vi "CenterBack.vi"(0 "Our Robot in":T3={"id"=0, "function"=enum."Attacker", "x"=0.0, "y"=0.0, "orientation"=0.0, "v_tangent"=0.0, "v_normal"=0.0, "v_ang"=0.0, "kick_x"=0.0, "kick_z"=0.0, "dribble"=FALSE, "Timestamp"=timestamp(0 s since 1904-01-01), "estimatives"={"est_v_tangent"=0.0, "est_v_normal"=0.0, "est_vx"=0.0, "est_vy"=0.0, "Pos Robot Est"=[]}, "dest_x_kick"=0.0, "dest_y_kick"=0.0, "Gap Coord"=[], "States"=enum."GoToTangent", "Path "=[], "Path  Smooth"=[], "Dest"=[]}, 1 "total":i32, 2 "Id duelist":u32, 3 "Stop?":bool, 4 "AI Parameters":T1={"GotoKick"={"Dist do cone a frente"=150.0, "attacker farback"=1500.0, "Perto"=300.0, "min dist to kick"=150.0, "kick eps"=0.05, "Time to transition"=0.0}, "Attacker"={"CC chute"=0.09, "CC passe"=0.045, "Kick Force"=100.0, "ball-robot Kick"=200.0, "ball-robot Pass"=0.3, "drible\nAttk"=FALSE}, "Defender"={"D max"=1700.0, "Vel p/ robô av"=1000.0, "Kick Force"=100.0, "D atk-def"=0.0, "D farback"=0.0, "drible\ndef"=FALSE, "drible\ngoalie"=FALSE}, "Timeout"={"Field/v in x"=6.0, "Dist Robots"=300, "Dist up in y"=300}, "Pose Striker"={"dist"=200.0, "Numeric"=-4.0, "dist 2"=200.0, "drible\nstriker"=FALSE}, "Dist Stop"=300.0, "D ball out"=200, "D central gap "=150.0, "T pass"=0.0, "Force ++"=0.0, "range kick"=0.0, "Chute alto"=TRUE, "Marcador novo"=TRUE, "drible"=FALSE, "D drible"=300.0, "Versão Striker"=enum."Auto", "Defesa"=enum."ManMark", "Marcador"=enum."Marcar Segundo mais perigoso", "Receptor passe"=enum."Auto", "Área"=enum."Quadrada", "Decisão\nsimples?"=FALSE} {"D drible" format="%#_13g"; "D central gap" format="%#_13g"; "Dist Stop" format="%#_13g"; "Pose Striker"."Numeric" format="%#_13g"; "Defender"."Kick Force" format="%#_13g"; "Defender"."Vel p/ robô av" format="%#_13g"; "Attacker"."ball-robot Kick" format="%#_13g"; "Attacker"."Kick Force" format="%#_13g"; "Attacker"."CC passe" format="%#_13g"; "Attacker"."CC chute" format="%#_13g"; "GotoKick"."kick eps" format="%#_13g"; "GotoKick"."min dist to kick" format="%#_13g"; "GotoKick"."Perto" format="%#_13g"; "GotoKick"."attacker farback" format="%#_13g"; "GotoKick"."Dist do cone a frente" format="%#_13g"}, 5 "balls":T8[](array[typedef]), 7 "Dribble":bool=TRUE, 9 "Field Size in":T9, 10 "Atacando contra?":bool=TRUE, 11 "Field defense":dbl[](array[numeric]), 12 "Defensores":u32[](array[numeric]), 14 "IA State Input 2":T2={"our_robots"=[], "enemy_robots"=[], "balls"=[], "geometry"={"line_width"=0, "field_length"=0, "field_width"=0, "boundary_width"=0, "referee_width"=0, "goal_width"=0, "goal_depth"=0, "goal_wall_width"=0, "center_circle_radius"=0, "defense_radius"=0, "defense_stretch"=0, "free_kick_from_defense_dist"=0, "penalty_spot_from_field_line_dist"=0, "penalty_line_from_spot_dist"=0}, "IA Judge"={"stage"="", "command"="", "our_goalie_id"=0.0, "enemy_goalie_id"=0.0, "command enum"=enum."Halt", "Time"=enum."Azul"}, "Received Timestamp"=timestamp(0 s since 1904-01-01), "Events"={"Touch"=FALSE, "Ball out"=FALSE, "id touch"=0.0, "Ball out of \nVision"=FALSE, "Ball inside \nGoalie area"=FALSE, "Robot not responding"=FALSE, "Robots responding status"=[1.0, 1.0, 1.0, 1.0, 1.0, 1.0], "Enemy Ball \nPossession"=FALSE, "Pass State"=FALSE, "id end of pass"=0.0, "Kick"=FALSE, "Id ini Possession"=0.0, "Ball Possesion"=FALSE, "Id Possesion"=0.0, "Direct Kick"=FALSE, "2nd Strk Ativo"=FALSE}}) -> (6 "Robot out":T3={"id"=0, "function"=enum."Attacker", "x"=0.0, "y"=0.0, "orientation"=0.0, "v_tangent"=0.0, "v_normal"=0.0, "v_ang"=0.0, "kick_x"=0.0, "kick_z"=0.0, "dribble"=FALSE, "Timestamp"=timestamp(0 s since 1904-01-01), "estimatives"={"est_v_tangent"=0.0, "est_v_normal"=0.0, "est_vx"=0.0, "est_vy"=0.0, "Pos Robot Est"=[]}, "dest_x_kick"=0.0, "dest_y_kick"=0.0, "Gap Coord"=[], "States"=enum."GoToTangent", "Path "=[], "Path  Smooth"=[], "Dest"=[]}, 8 "Pos Centers Back":dbl[][](array[numeric]), 13 "Zageuiro duelist?":bool=TRUE)   [LabVIEW 2018]
uses:
  Core/AI Robot.ctl
  Functions Enum.ctl
  AttackerStates.ctl
  Path Planning/RRT/PathDests.ctl
  Path Planning/RRT/PathDest.ctl
  Core/AI Ball.ctl
  Core/Field Size.ctl
  Core/AI Input.ctl
  Core/AI Judge.ctl
  Command Enum.ctl
  Util/Events/Events.ctl
  AI Parameters.ctl
  PersonalityEnum.ctl
  <vilib>/Analysis/_algsub.llb/Real Vector Norm.vi
  <vilib>/Analysis/NI_AALPro.lvlib
panel:
  in  "element":dbl=-2000.0 format="%#_13g"
  in  "dist to defender\nattacker evasion":dbl=200.0
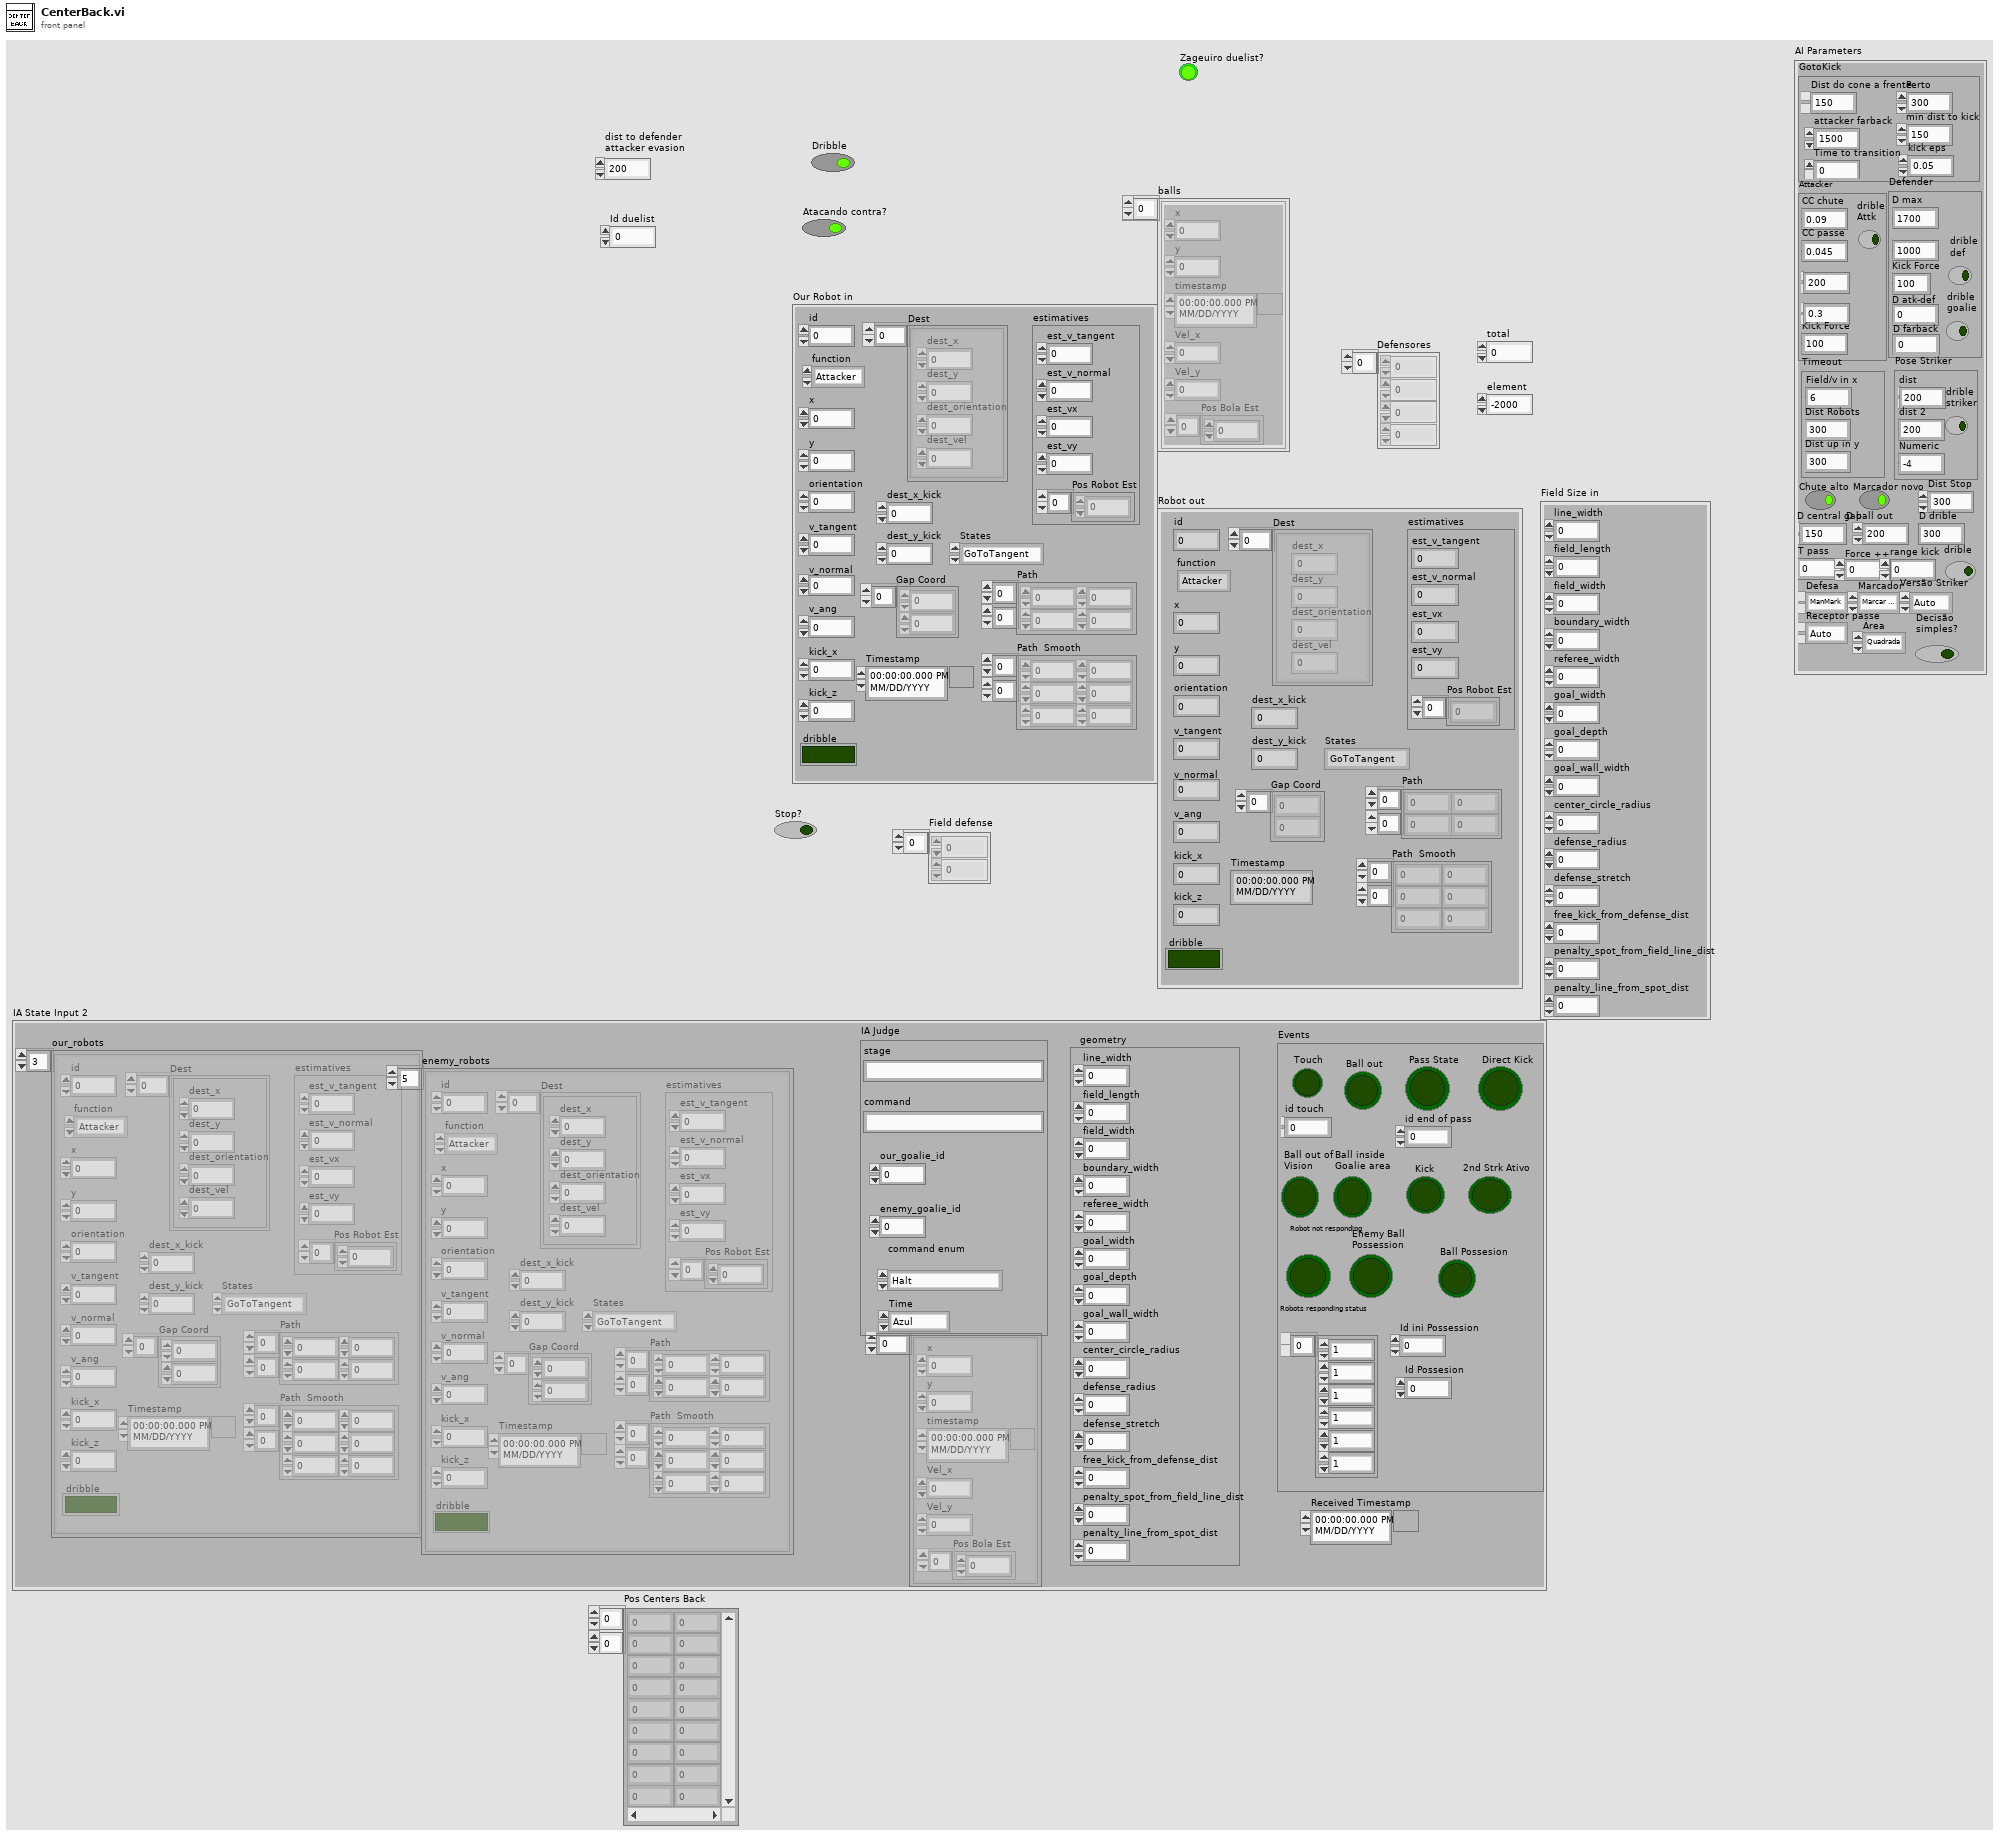
[diagram p1: front panel]
types:
  T1 = typedef "AI Parameters.ctl" = cluster{"GotoKick":cluster{"Dist do cone a frente":dbl, "attacker farback":dbl, "Perto":dbl, "min dist to kick":dbl, "kick eps":dbl, "Time to transition":dbl}, "Attacker":cluster{"CC chute":dbl, "CC passe":dbl, "Kick Force":dbl, "ball-robot Kick":dbl, "ball-robot Pass":dbl, "drible\nAttk":bool}, "Defender":cluster{"D max":dbl, "Vel p/ robô av":dbl, "Kick Force":dbl, "D atk-def":dbl, "D farback":dbl, "drible\ndef":bool, "drible\ngoalie":bool}, "Timeout":cluster{"Field/v in x":dbl, "Dist Robots":u32, "Dist up in y":u32}, "Pose Striker":cluster{"dist":dbl, "Numeric":dbl, "dist 2":dbl, "drible\nstriker":bool}, "Dist Stop":dbl, "D ball out":i32, "D central gap ":dbl, "T pass":dbl, "Force ++":dbl, "range kick":dbl, "Chute alto":bool, "Marcador novo":bool, "drible":bool, "D drible":dbl, "Versão Striker":enum16{"Auto", "3", "2", "1"}, "Defesa":enum16{"ManMark", "Barreira"}, "Marcador":enum16{"Marcar Segundo mais perigoso", "Marcar o mais perigoso"}, "Receptor passe":enum16{"Auto", "2nd Striker", "Striker"}, "Área":enum16{"Quadrada", "Circular"}, "Decisão\nsimples?":bool}
  T2 = typedef "AI Input.ctl" = cluster{"our_robots":T3[], "enemy_robots":T3[], "balls":T8[], "geometry":T9, "IA Judge":T10, "Received Timestamp":timestamp, "Events":T12}
  T3 = typedef "AI Robot.ctl" = cluster{"id":u32, "function":T4, "x":dbl, "y":dbl, "orientation":dbl, "v_tangent":dbl, "v_normal":dbl, "v_ang":dbl, "kick_x":dbl, "kick_z":dbl, "dribble":bool, "Timestamp":timestamp, "estimatives":cluster{"est_v_tangent":dbl, "est_v_normal":dbl, "est_vx":dbl, "est_vy":dbl, "Pos Robot Est":dbl[]}, "dest_x_kick":dbl, "dest_y_kick":dbl, "Gap Coord":dbl[], "States":T5, "Path ":dbl[][], "Path  Smooth":dbl[][], "Dest":T6}
  T4 = typedef "Functions Enum.ctl" = enum16{"2nd Striker", "Attacker", "Goalie", "Defender", "Striker", "Goto 0", "Dummy", "Kicker", "ZigZag 0", "ZigZag 1", "ZigZag 2", "ZigZag 3", "ZigZag 4", "ZigZag 5", "ZigZag 6", "ZigZag 7", "ZigZag 8", ""}
  T5 = typedef "AttackerStates.ctl" = enum16{"Pass", "GoToTangent", "BallGetting", "GoToKick", ""}
  T6 = typedef "PathDests.ctl" = T7[]
  T7 = typedef "PathDest.ctl" = cluster{"dest_x":dbl, "dest_y":dbl, "dest_orientation":dbl, "dest_vel":dbl}
  T8 = typedef "AI Ball.ctl" = cluster{"x":dbl, "y":dbl, "timestamp":timestamp, "Vel_x":dbl, "Vel_y":dbl, "Pos Bola Est":dbl[]}
  T9 = typedef "Field Size.ctl" = cluster{"line_width":u32, "field_length":u32, "field_width":u32, "boundary_width":u32, "referee_width":u32, "goal_width":u32, "goal_depth":u32, "goal_wall_width":u32, "center_circle_radius":u32, "defense_radius":u32, "defense_stretch":u32, "free_kick_from_defense_dist":u32, "penalty_spot_from_field_line_dist":u32, "penalty_line_from_spot_dist":u32}
  T10 = typedef "AI Judge.ctl" = cluster{"stage":string, "command":string, "our_goalie_id":dbl, "enemy_goalie_id":dbl, "command enum":T11, "Time":enum16{"Azul", "Amarelo"}}
  T11 = typedef "Command Enum.ctl" = enum16{"Halt", "Stop", "Force Start", "PKA Normal Start", "Prepare Kickoff Ally", "PKE Normal Start", "Prepare Kickoff Enemy", "Prepare Penalty Ally", "PPA Normal Start", "Prepare Penalty Enemy", "PPE Normal Start", "Direct Free Enemy", "Direct Free Ally", "Indirect Free Enemy", "Indirect Free Ally", "Timeout Enemy", "Timeout Ally", "Goal Enemy", "Goal Ally", "Ball Placement Enemy", "Ball Placement Ally", "Normal Half Time", "Extra Time Break", "Extra Half Time", "None", "Post Game"}
  T12 = typedef "Events.ctl" = cluster{"Touch":bool, "Ball out":bool, "id touch":dbl, "Ball out of \nVision":bool, "Ball inside \nGoalie area":bool, "Robot not responding":bool, "Robots responding status":dbl[], "Enemy Ball \nPossession":bool, "Pass State":bool, "id end of pass":dbl, "Kick":bool, "Id ini Possession":dbl, "Ball Possesion":bool, "Id Possesion":dbl, "Direct Kick":bool, "2nd Strk Ativo":bool}
  T13 = cluster{"D max":dbl, "Vel p/ robô av":dbl, "Kick Force":dbl, "D atk-def":dbl, "D farback":dbl, "drible\ndef":bool, "drible\ngoalie":bool}
  T14 = typedef "PersonalityEnum.ctl" = enum16{"Attacker", "Striker", "Defender", "Goalie"}
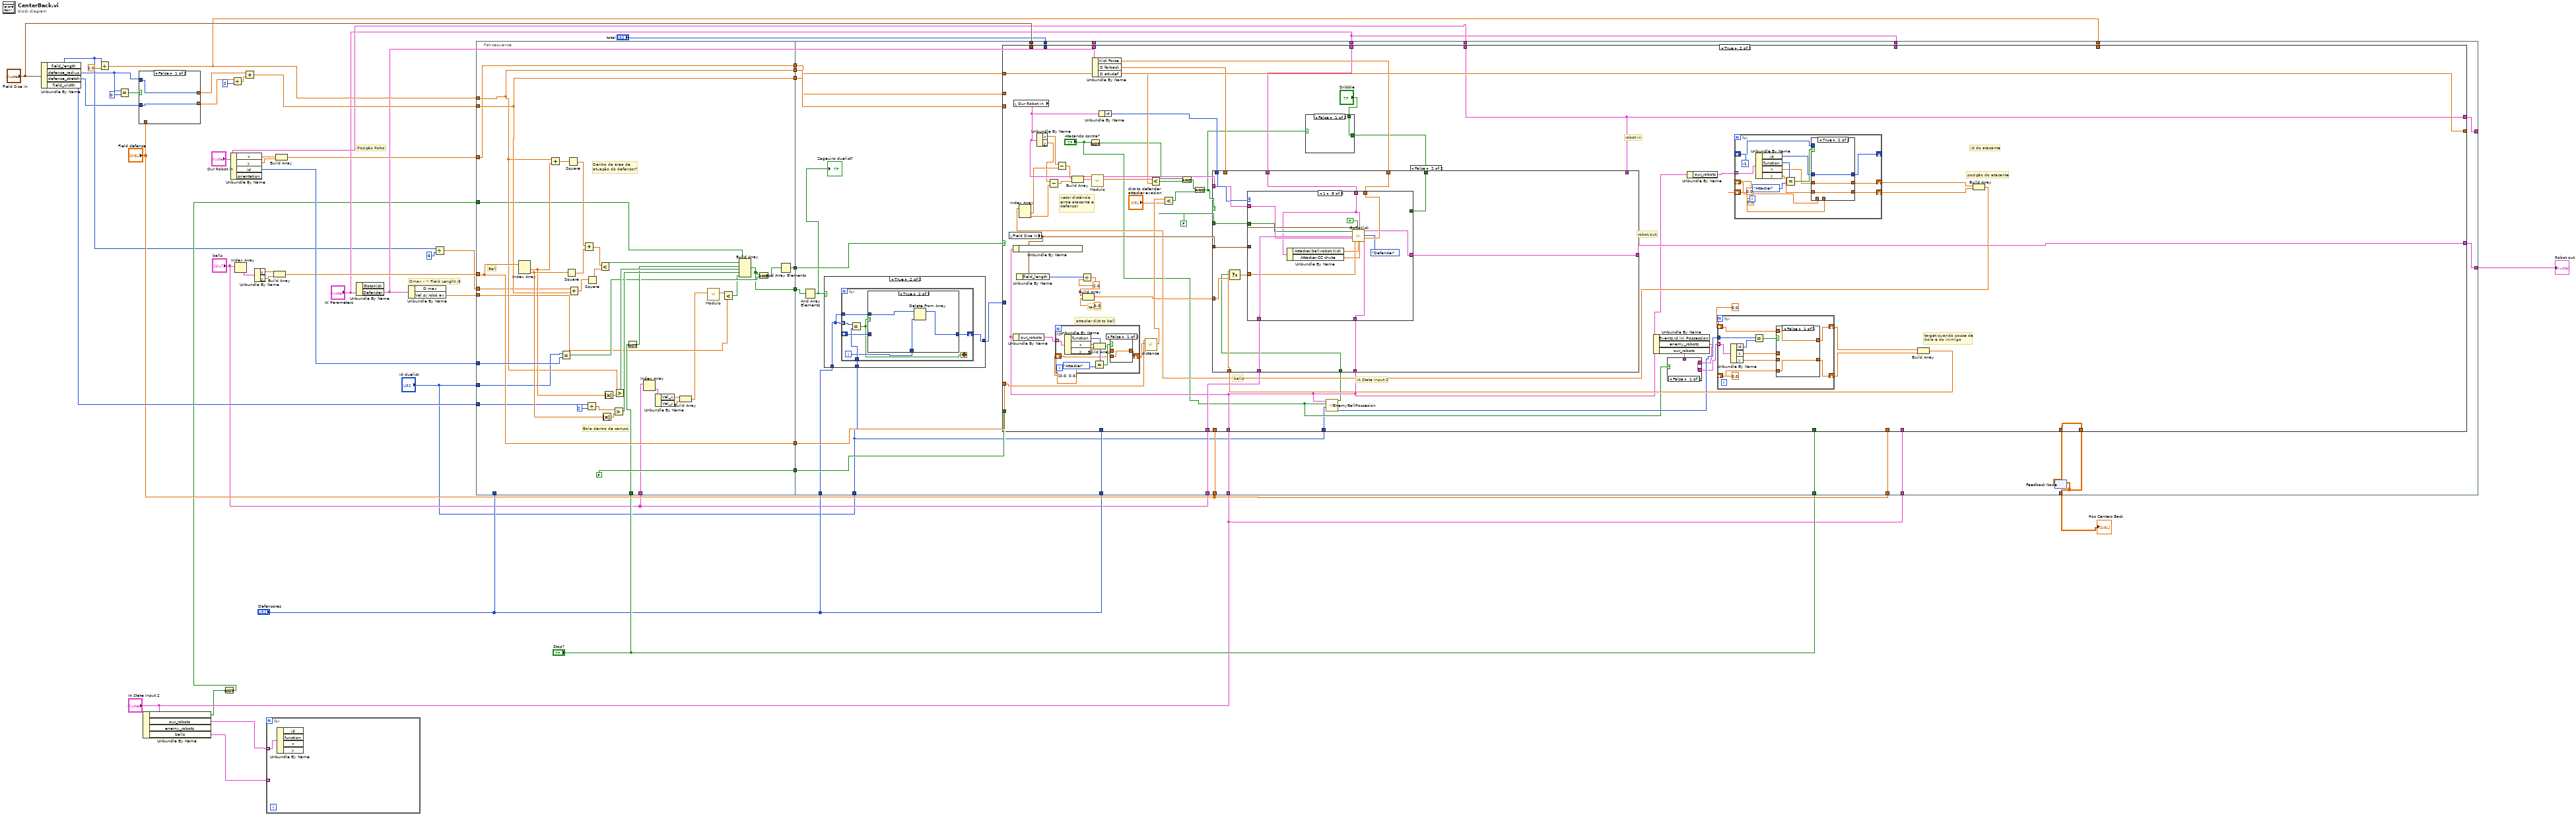
[diagram p0: block diagram]
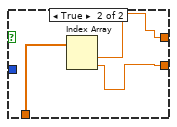
[diagram p2: hidden frame]
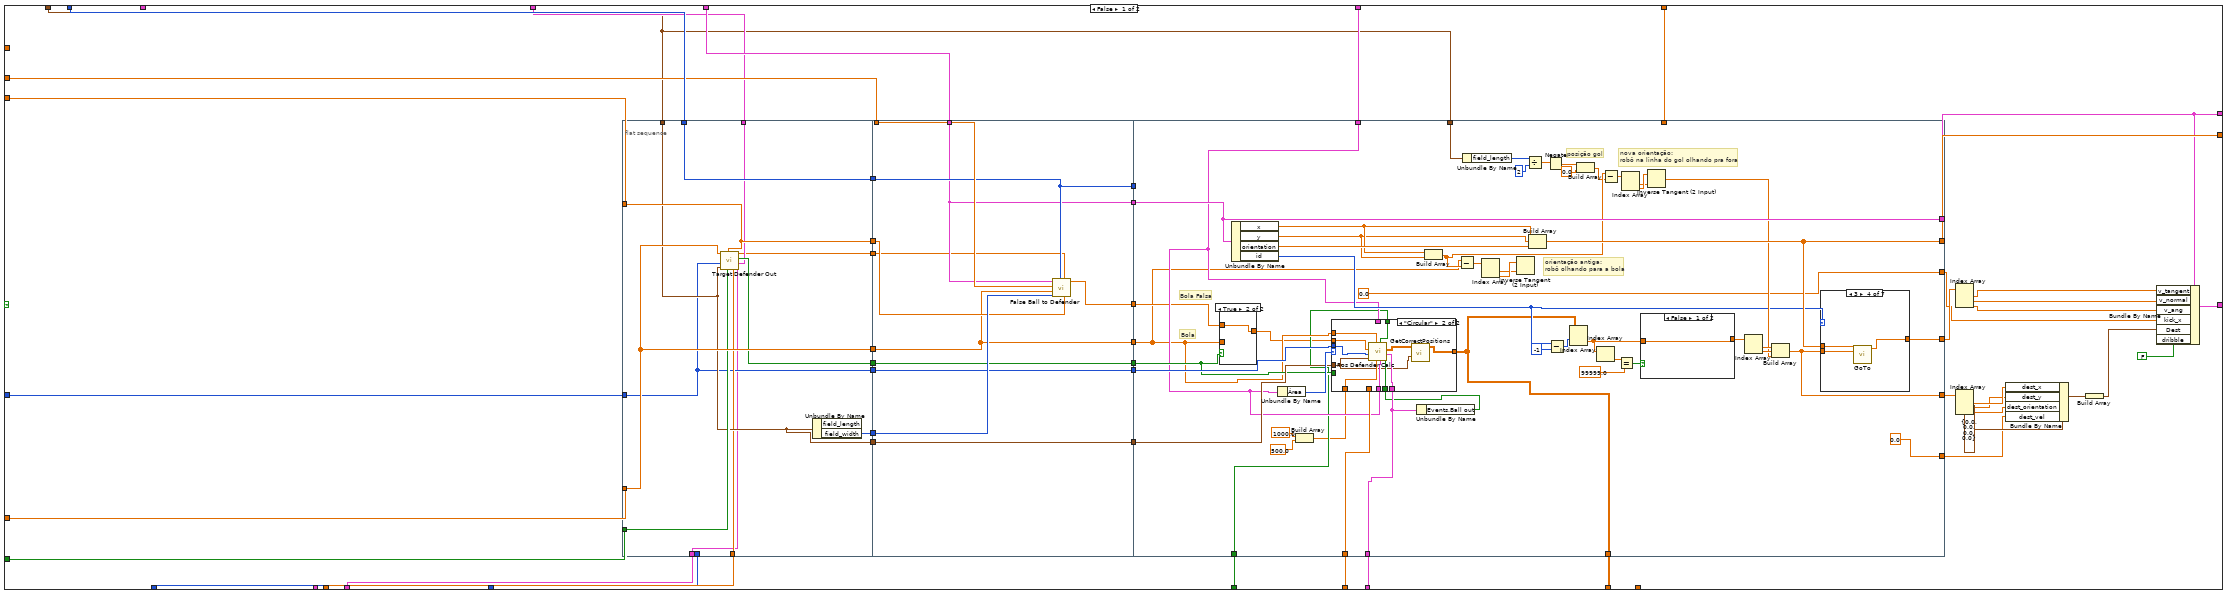
[diagram p5: hidden frame]
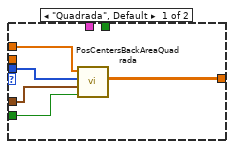
[diagram p6: hidden frame]
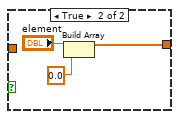
[diagram p7: hidden frame]
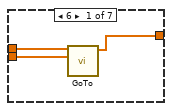
[diagram p8: hidden frame]
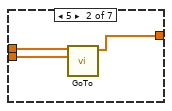
[diagram p9: hidden frame]
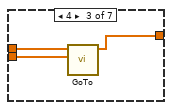
[diagram p10: hidden frame]
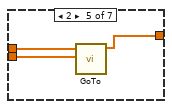
[diagram p11: hidden frame]
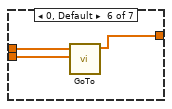
[diagram p12: hidden frame]
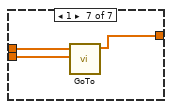
[diagram p13: hidden frame]
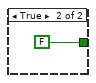
[diagram p15: hidden frame]
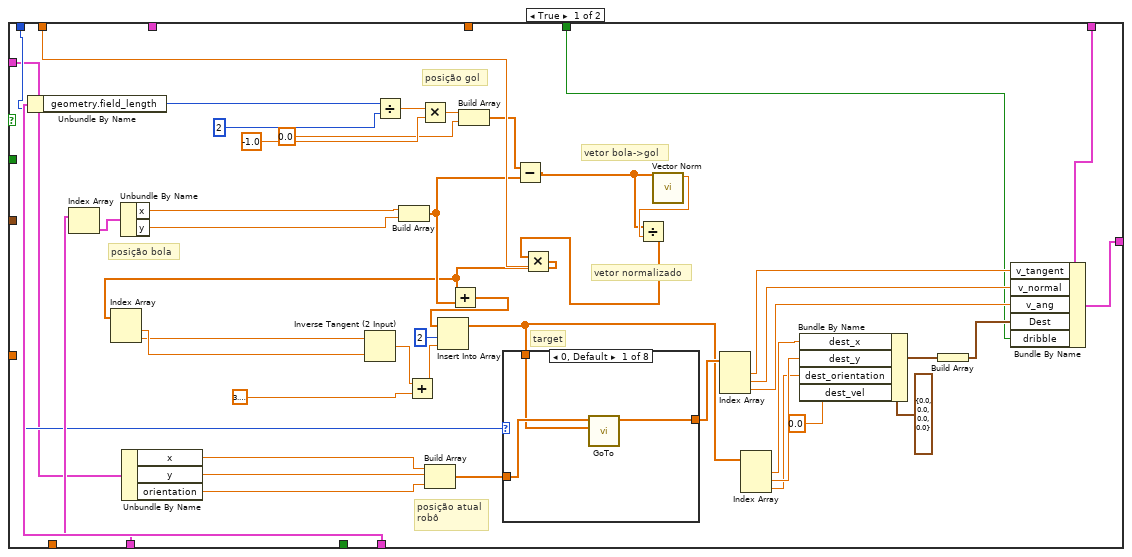
[diagram p18: hidden frame]
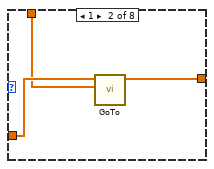
[diagram p19: hidden frame]
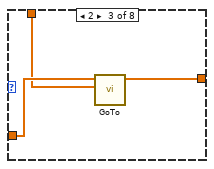
[diagram p20: hidden frame]
diagram:
  # "Dmax - > Field Lenght /6"
  # "Posição Robo"
  n1 = Unbundle By Name("Field Size in") -> ("field_length"=w3:u32, "defense_radius"=w28:u32, "defense_stretch"=w27:u32, "field_width"=w41:u32)
  n2 = Divide(x=w3, y=2.0) -> (x/y=w19:dbl)
  n3 = Equal?(x=w28, y=u32 0) -> (x = y?=w26:bool)
  n4 = case shown="False" w26 {
    tunnel: [w50 w52] -> w25
    tunnel: w28 -> [w50 _]
    tunnel: w27 -> [w49 _]
    tunnel: [w49 w51] -> w24
    tunnel: "Field defense" -> [_ w53]
    frame False {
    }
    frame True {
      n5 = Index Array(array=w53) -> (element #1=w52:dbl, element #2=w51:dbl)  [unwired: 2 in]
    }
  }
  n6 = Unbundle By Name("IA State Input 2") -> ("Events.Ball inside \nGoalie area"=w5:bool, "our_robots"=w10:T3[], "balls"=w9:T8[])  [unwired: 1 out]
  n7 = Not(x=w5) -> (.not. x?=w4:bool)
  n8 = Unbundle By Name("Our Robot in") -> ("x"=w38:dbl, "y"=w37:dbl, "id"=w42:u32)  [unwired: 1 out]
  n9 = Divide(x=w24, y=u32 2) -> (x/y=w47:dbl)
  n10 = Index Array(array="balls") -> (element=w48:T8)  [unwired: 1 in]
  n11 = Add(x=w25, y=w47) -> (x+y=w43:dbl)
  n12 = Unbundle By Name(w48) -> ("x"=w45:dbl, "y"=w12:dbl)
  n13 = for {
    tunnel: w10 -> [w54] mode=indexing
    tunnel: w9 -> [_] mode=indexing
    n14 = Unbundle By Name(w54) -> ()  [unwired: 4 out]
  }
  n15 = Build Array(w45, w12) -> (w20:dbl[])
  n16 = Build Array(w38, w37) -> (w21:dbl[])
  n17 = Unbundle By Name("AI Parameters") -> ("Defender"=w14:T13)  [unwired: 1 out]
  n18 = Unbundle By Name(w14) -> ("Vel p/ robô av"=w15:dbl)  [unwired: 1 out]
  n19 = Divide(x=w3, y=u32 6) -> (x/y=w1:dbl)
  n20 = flat-sequence {
    tunnel: w43 -> [w73]
    tunnel: w19 -> [w72]
    tunnel: w20 -> [w88]
    tunnel: w21 -> [w71]
    tunnel: [w88] -> w36
    tunnel: [w93] -> w35
    tunnel: w42 -> [w92]
    tunnel: w41 -> [w79]
    tunnel: [FALSE ("Target Fora")] -> w34
    tunnel: [w72] -> w33
    tunnel: [w73] -> w32
    tunnel: [w71] -> w31
    tunnel: "Defensores" -> [_]
    tunnel: "Stop?" -> [w70]
    tunnel: [w66] -> w17
    tunnel: "balls" -> [w65]
    tunnel: w1 -> [w62]
    tunnel: w15 -> [w61]
    tunnel: "Id duelist" -> [w56]
    tunnel: w4 -> [w55]
    tunnel: "total" -> [w122]
    tunnel: [w121] -> w8
    tunnel: w36 -> [w120]
    tunnel: w35 -> [w119]
    tunnel: w34 -> [w118]
    tunnel: w33 -> [w116]
    tunnel: "Field Size in" -> [w117]
    tunnel: "Our Robot in" -> [w115]
    tunnel: w32 -> [w114]
    tunnel: [w113] -> _
    tunnel: w31 -> [w112]
    tunnel: "Field defense" -> [w111]
    tunnel: "Field defense" -> [w110]
    tunnel: "Defensores" -> [w109]
    tunnel: "IA State Input 2" -> [w108]
    tunnel: "balls" -> [w107]
    tunnel: "Stop?" -> [w106]
    tunnel: w19 -> [w105]
    tunnel: "Defensores" -> [w104]
    tunnel: w17 -> [w103]
    tunnel: w14 -> [w101]
    tunnel: "AI Parameters" -> [w100]
    tunnel: "AI Parameters" -> [w99]
    tunnel: "IA State Input 2" -> [w98]
    tunnel: [w95] -> w7
    tunnel: "Id duelist" -> [w94]
    frame #0 {
      # "Bola dentro de campo"
      # "Dentro da área de \natuação do defensor?"
      # "Ball"
      n21 = Index Array(array=w88) -> (element #1=w76:dbl, element #2=w80:dbl)  [unwired: 2 in]
      n22 = Add(x=w72, y=w76) -> (x+y=w89:dbl)
      n23 = Equal?(x=w56, y=w92) -> (x = y?=w68:bool)
      n24 = Square(x=w80) -> (x^2=w91:dbl)
      n25 = Square(x=w89) -> (x^2=w90:dbl)
      n26 = Add(x=w62, y=w73) -> (x+y=w75:dbl)
      n27 = Add(x=w90, y=w91) -> (x+y=w85:dbl)
      n28 = Divide(x=w79, y=u32 2) -> (x/y=w82:dbl)
      n29 = Square(x=w75) -> (x^2=w87:dbl)
      n30 = Less?(x=w85, y=w87) -> (x < y?=w86:bool)
      n31 = Absolute Value(x=w80) -> (abs(x)=w81:dbl)
      n32 = Absolute Value(x=w76) -> (abs(x)=w84:dbl)
      n33 = Greater?(x=w82, y=w81) -> (0:w77:bool)
      n34 = Greater?(x=w72, y=w84) -> (0:w83:bool)
      n35 = Not(x=w70) -> (.not. x?=w69:bool)
      n36 = Index Array(array=w65) -> (element=w60:T8)  [unwired: 1 in]
      n37 = Unbundle By Name(w60) -> ("Vel_x"=w59:dbl, "Vel_y"=w58:dbl)
      n38 = Build Array(w59, w58) -> (w57:dbl[])
      n39 = call "Modulo.vi"("2D vector"=w57) -> ("Modulo"=w63:dbl)  [unwired: 10 in]
      n40 = Less?(x=w63, y=w61) -> (x < y?=w64:bool)
      n41 = Build Array(w55, w86, w69, w83, w77, w64) -> (w66:bool[])
      n42 = And(x=w66, y=w68) -> (x .and. y?=w67:bool[])
      n43 = And Array Elements(Boolean array=w67) -> (logical AND=w93:bool)
    }
    frame #1 {
      n44 = And Array Elements(Boolean array=w103) -> (logical AND=w97:bool)
      "Zageuiro duelist?" <- w97
      n45 = case shown="True" w97 {
        tunnel: w104 -> [w123 w125]
        tunnel: [w123 w124] -> w102
        tunnel: w94 -> [_ w126]
        frame False {
        }
        frame True {
          n46 = for {
            tunnel: w125 -> [w133] mode=indexing
            tunnel: w126 -> [w132]
            tunnel: w125 -> [w131]
            shift-right: [w129] -> w124
            shift-left: _ -> [w128]
            i -> [w130]
            stop <- w127 stop-if-true
            n47 = Equal?(x=w133, y=w132) -> (x = y?=w127:bool)
            n48 = case shown="True" w127 {
              tunnel: w131 -> [_ w137]
              tunnel: w130 -> [_ w136]
              tunnel: [w134 w135] -> w129
              tunnel: w128 -> [w134 _]
              frame False {
              }
              frame True {
                n49 = Delete From Array(array=w137, index=w136) -> (array with subset deleted=w135:u32[])  [unwired: 1 in, 1 out]
              }
            }
          }
        }
      }
      n50 = feedback #1() -> (w95:dbl[][])  [unwired: 1 in]
      n51 = case shown="True" w119 {
        tunnel: w122 -> [w186 _]
        tunnel: [w182 w328] -> w121
        tunnel: w120 -> [w181 w321]
        tunnel: w118 -> [w179 _]
        tunnel: w116 -> [w178 _]
        tunnel: w117 -> [w148 _]
        tunnel: w115 -> [w177 w329]
        tunnel: w114 -> [w176 _]
        tunnel: [w162 w363] -> _
        tunnel: [w161 w329] -> w113
        tunnel: w112 -> [_ w363]
        tunnel: w111 -> [w160 _]
        tunnel: w110 -> [w159 _]
        tunnel: w109 -> [w158 _]
        tunnel: w108 -> [w151 w315]
        tunnel: w107 -> [_ w362]
        tunnel: w106 -> [w157 _]
        tunnel: w105 -> [w156 _]
        tunnel: w102 -> [w154 _]
        tunnel: w101 -> [_ w348]
        tunnel: w100 -> [w150 w346]
        tunnel: w99 -> [w153 _]
        tunnel: w98 -> [w152 _]
        tunnel: [w141 w316] -> w96
        tunnel: w95 -> [_ w316]
        tunnel: w94 -> [_ w307]
        frame False {
          n52 = flat-sequence {
            tunnel: w186 -> [w198]
            tunnel: [w199] -> w187
            tunnel: w181 -> [w197]
            tunnel: [w198] -> w180
            tunnel: w179 -> [w195]
            tunnel: w178 -> [w196]
            tunnel: w148 -> [w193]
            tunnel: [w197] -> w175
            tunnel: [w196] -> w174
            tunnel: [w194] -> w170
            tunnel: [w191] -> w167
            tunnel: [w193] -> w165
            tunnel: w159 -> [w192]
            tunnel: w158 -> [_]
            tunnel: w154 -> [w191]
            tunnel: w151 -> [w190]
            tunnel: w150 -> [w189]
            tunnel: [w188] -> w149
            tunnel: w187 -> [w210]
            tunnel: w180 -> [w205]
            tunnel: w177 -> [w202]
            tunnel: w176 -> [w209]
            tunnel: w175 -> [w207]
            tunnel: w174 -> [w208]
            tunnel: [w200] -> w173
            tunnel: [w207] -> w172
            tunnel: [w206] -> w171
            tunnel: w170 -> [w206]
            tunnel: [w205] -> w169
            tunnel: [w204] -> w168
            tunnel: w167 -> [w204]
            tunnel: [w203] -> w166
            tunnel: w165 -> [w203]
            tunnel: [w202] -> w164
            tunnel: w149 -> [w201]
            tunnel: [w254] -> w163
            tunnel: [w253] -> w161
            tunnel: w173 -> [w219]
            tunnel: w172 -> [w218]
            tunnel: w171 -> [w221]
            tunnel: w169 -> [_]
            tunnel: w168 -> [w222]
            tunnel: w166 -> [w223]
            tunnel: w164 -> [w253]
            tunnel: [w250] -> w162
            tunnel: w160 -> [w224]
            tunnel: w157 -> [w215]
            tunnel: w156 -> [_]
            tunnel: [w244] -> w155
            tunnel: w153 -> [w220]
            tunnel: w152 -> [w217]
            tunnel: w148 -> [w243]
            tunnel: [w225] -> w141
            tunnel: [0.0 ("dest_vel")] -> w140
            tunnel: [0.0 ("kick_x")] -> w139
            frame #0 {
              n53 = call "Target Defender Out.vi"("IA State Input"=w190, "AI Parameters"=w189, "Field defense"=w192, "Target Fora in"=w195, "Campo/2"=w196, "Field Size in"=w193, "Defensores"=w191, "Ball"=w197) -> ("Target Fora out"=w194:bool, "Central Position"=w188:dbl[])  [unwired: 2 in]
              n54 = Unbundle By Name(w193) -> ("field_width"=w199:u32)  [unwired: 1 out]
            }
            frame #1 {
              n55 = call "False Ball to Defender.vi"("Campo/2"=w208, "Central Position"=w201, "field_width"=w210, "total"=w205, "Bola"=w207, "raio da área \ndo goleiro"=w209, "Our Robot in"=w202) -> ("Bola Falsa"=w200:dbl[])  [unwired: 4 in]
            }
            frame #2 {
              # "nova orientação:\nrobô na linha do gol olhando pra fora"
              # "orientação antiga:\nrobô olhando para a bola"
              # "posição gol"
              # "Bola"
              # "Bola Falsa"
              n56 = case shown="True" w221 {
                tunnel: [w302 w303] -> w211
                tunnel: w218 -> [w302 _]
                tunnel: w219 -> [_ w303]
                frame False {
                }
                frame True {
                }
              }
              n57 = Unbundle By Name(w253) -> ("x"=w259:dbl, "y"=w258:dbl, "orientation"=w260:dbl, "id"=w229:u32)
              n58 = Unbundle By Name(w220) -> ("Área"=w226:enum16{"Quadrada", "Circular"})
              n59 = Build Array(1000.0, 500.0) -> (w212:dbl[])
              n60 = Unbundle By Name(w217) -> ("Events.Ball out"=w216:bool)
              n61 = case shown="\"Circular\"" w226 {
                tunnel: [w265 w269] -> w225
                tunnel: w224 -> [_ _]
                tunnel: w217 -> [_ w276]
                tunnel: w223 -> [w264 w266]
                tunnel: w222 -> [w263 w273]
                tunnel: w218 -> [w262 w274]
                tunnel: w221 -> [w261 _]
                tunnel: w220 -> [_ _]
                tunnel: w220 -> [_ w275]
                tunnel: w216 -> [_ w272]
                tunnel: w215 -> [_ w271]
                tunnel: w212 -> [_ w268]
                tunnel: w211 -> [_ w267]
                frame "Quadrada", Default {
                  n62 = call "PosCentersBackAreaQuadrada.vi"("Robô fora?"=w261, "geometry"=w264, "Defensores"=w263, "Pos Bola"=w262) -> ("Pos Centers Back"=w265:dbl[][])  [unwired: 6 in, 1 out]
                }
                frame "Circular" {
                  n63 = call "Pos Defender Calc.vi"("Events.Ball out"=w272, "IA State Input"=w276, "AI Parameters"=w275, "Stop?"=w271, "Field defense"=w268, "Real Ball"=w274, "Field Size in"=w266, "Defensores"=w273, "Ball"=w267) -> ("Posição dos Defensores"=w270:dbl[][])  [unwired: 1 in, 1 out]
                  n64 = call "GetCorrectPositions.vi"("Field Size in"=w266, "Posição dos defensores"=w270) -> ("Posição dos defensores correta"=w269:dbl[][])  [unwired: 9 in]
                }
              }
              n65 = Build Array(w259, w258) -> (w237:dbl[])
              n66 = Subtract(x=w218, y=w237) -> (x-y=w257:dbl[])
              n67 = Unbundle By Name(w243) -> ("field_length"=w242:u32)
              n68 = Index Array(array=w257) -> (element #1=w255:dbl, element #2=w256:dbl)  [unwired: 2 in]
              n69 = Inverse Tangent (2 Input)(1:w255, 2:w256) -> ()  [unwired: 1 out]
              n70 = Divide(x=w242, y=u32 2) -> (x/y=w240:dbl)
              n71 = Build Array(w259, w258, w260) -> (w250:dbl[])
              n72 = Negate(x=w240) -> (-x=w239:dbl)
              n73 = Subtract(x=w229, y=-1) -> (x-y=w227:u32)
              n74 = Index Array(array=w225, index (row)=w227) -> (element=w248:dbl[])  [unwired: 1 in]
              n75 = Build Array(w239, 0.0 ("element")) -> (w236:dbl[])
              n76 = Index Array(array=w248) -> (element=w247:dbl)  [unwired: 1 in]
              n77 = Subtract(x=w237, y=w236) -> (x-y=w235:dbl[])
              n78 = Equal?(x=w247, y=99999.0) -> (x = y?=w246:bool)
              n79 = Index Array(array=w235) -> (element #1=w233:dbl, element #2=w234:dbl)  [unwired: 2 in]
              n80 = case shown="False" w246 {
                tunnel: [w277 w279] -> w249
                tunnel: w248 -> [w277 _]
                frame False {
                }
                frame True {
                  n81 = Build Array("element", 0.0 ("element")) -> (w279:dbl[])
                }
              }
              n82 = Inverse Tangent (2 Input)(1:w233, 2:w234) -> (0:w232:dbl)
              n83 = Index Array(array=w249) -> (element #1=w252:dbl, element #2=w251:dbl)  [unwired: 2 in]
              n84 = Build Array(w252, w251, w232) -> (w244:dbl[])
              n85 = case shown="3" w229 {
                tunnel: [w281 w284 w287 w290 w293 w296 w299] -> w254
                tunnel: w244 -> [w282 w286 w288 w291 w294 w297 w300]
                tunnel: w250 -> [w283 w285 w289 w292 w295 w298 w301]
                frame 6 {
                  n86 = call "GoTo.vi"("Target"=w282, "Position"=w283) -> ("Output\nVelocity"=w281:dbl[])  [unwired: 8 in, 1 out]
                }
                frame 5 {
                  n87 = call "GoTo.vi"("Target"=w286, "Position"=w285) -> ("Output\nVelocity"=w284:dbl[])  [unwired: 8 in, 1 out]
                }
                frame 4 {
                  n88 = call "GoTo.vi"("Target"=w288, "Position"=w289) -> ("Output\nVelocity"=w287:dbl[])  [unwired: 8 in, 1 out]
                }
                frame 3 {
                  n89 = call "GoTo.vi"("Target"=w291, "Position"=w292) -> ("Output\nVelocity"=w290:dbl[])  [unwired: 8 in, 1 out]
                }
                frame 2 {
                  n90 = call "GoTo.vi"("Target"=w294, "Position"=w295) -> ("Output\nVelocity"=w293:dbl[])  [unwired: 8 in, 1 out]
                }
                frame 0, Default {
                  n91 = call "GoTo.vi"("Target"=w297, "Position"=w298) -> ("Output\nVelocity"=w296:dbl[])  [unwired: 8 in, 1 out]
                }
                frame 1 {
                  n92 = call "GoTo.vi"("Target"=w300, "Position"=w301) -> ("Output\nVelocity"=w299:dbl[])  [unwired: 8 in, 1 out]
                }
              }
            }
          }
          n93 = Index Array(array=w163) -> (element #1=w185:dbl, element #2=w184:dbl, element #3=w183:dbl)  [unwired: 3 in]
          n94 = Index Array(array=w155) -> (element #1=w144:dbl, element #2=w143:dbl, element #3=w142:dbl)  [unwired: 3 in]
          n95 = Bundle By Name(cluster=T7 {"dest_x"=0.0, "dest_y"=0.0, "dest_orientation"=0.0, "dest_vel"=0.0} ("Dest"), "dest_x"=w144, "dest_y"=w143, "dest_orientation"=w142, "dest_vel"=w140) -> (w146:T7)
          n96 = Build Array(w146) -> (w145:T7[])
          n97 = Bundle By Name(cluster=w161, "v_tangent"=w185, "v_normal"=w184, "v_ang"=w183, "kick_x"=w139, "Dest"=w145, "dribble"=FALSE) -> (w182:T3)
        }
        frame True {
          # "attacker dist to ball"
          # "robot in"
          # "vetor distância\nentre atacante e \ndefensor"
          # "posição do atacante"
          # "id do atacante"
          # "target quando posse de\nbola é do inimigo"
          # "target"
          # "balls"
          # "IA State Input 2"
          # "robot out"
          n98 = local read "Field Size in"() -> (w358:T9)
          n99 = Unbundle By Name(w315) -> ()  [unwired: 1 out]
          n100 = Unbundle By Name(w315) -> ("our_robots"=w324:T3[])
          n101 = local read "Our Robot in"() -> (w339:T3)
          n102 = Unbundle By Name(w358) -> ("field_length"=w357:u32)
          n103 = Unbundle By Name(w339) -> ("x"=w337:dbl, "y"=w335:dbl)
          n104 = for {
            tunnel: w324 -> [w376] mode=indexing
            shift-right: [w370] -> w322
            shift-left: dbl[] [0.0, 0.0] -> [w369]
            n105 = Unbundle By Name(w376) -> ("function"=w375:T4, "x"=w368:dbl, "y"=w372:dbl)
            n106 = Build Array(w368, w372) -> (w371:dbl[])
            n107 = Equal?(x=w375, y=Functions_Enum."Attacker") -> (x = y?=w373:bool)
            n108 = case shown="False" w373 {
              tunnel: w371 -> [_ w378]
              tunnel: [w377 w378] -> w370
              tunnel: w369 -> [w377 _]
              frame False {
              }
              frame True {
              }
            }
          }
          n109 = Divide(x=w357, y=2.0) -> (x/y=w355:dbl)
          n110 = Build Array(w355, 0.0) -> (w360:dbl[])
          n111 = Not(x="Atacando contra?") -> (.not. x?=w312:bool)
          n112 = Unbundle By Name(w348) -> ("Kick Force"=w347:dbl, "D farback"=w326:dbl, "D atk-def"=w327:dbl)
          n113 = Unbundle By Name(w339) -> ("id"=w361:u32)
          n114 = call "distance.vi"("P1"=w322, "P2"=w321) -> ("Dist P1P2"=w320:dbl)  [unwired: 9 in]
          n115 = Less?(x=w320, y="dist to defender\nattacker evasion") -> (x < y?=w318:bool)
          n116 = call "EnemyBallPossesion.vi"("Id Duelist"=w307, "Atacando contra?"="Atacando contra?", "IA State Input"=w315) -> ("Id Enemy Ball Possesion"=w314:u32, "Enemy Ball Possesion?"=w313:bool)  [unwired: 7 in]
          n117 = Unbundle By Name(w315) -> ("enemy_robots"=w308:T3[], "our_robots"=w309:T3[])  [unwired: 1 out]
          n118 = case shown="False" "Atacando contra?" {
            tunnel: [w366 w367] -> w310
            tunnel: w309 -> [_ w367]
            tunnel: w308 -> [w366 _]
            frame False {
            }
            frame True {
            }
          }
          n119 = Unbundle By Name(w315) -> ("our_robots"=w345:T3[])
          n120 = for {
            tunnel: w310 -> [w595] mode=indexing
            tunnel: w314 -> [w593]
            shift-right: [w589] -> w353
            shift-left: 0.0 ("x") -> [w587]
            shift-right: [w588] -> w352
            shift-left: 0.0 ("y") -> [w586]
            n121 = Unbundle By Name(w595) -> ("id"=w594:u32, "x"=w591:dbl, "y"=w590:dbl)
            n122 = Equal?(x=w593, y=w594) -> (x = y?=w592:bool)
            n123 = case shown="False" w592 {
              tunnel: w591 -> [_ w599]
              tunnel: w590 -> [_ w598]
              tunnel: [w597 w599] -> w589
              tunnel: [w596 w598] -> w588
              tunnel: w587 -> [w597 _]
              tunnel: w586 -> [w596 _]
              frame False {
              }
              frame True {
              }
            }
          }
          n124 = for {
            tunnel: w345 -> [w579] mode=indexing
            shift-right: [w572] -> _
            shift-left: -1 -> [w571]
            shift-right: [w570] -> w341
            shift-left: 0.0 ("y") -> [w568]
            shift-right: [w569] -> w340
            shift-left: 0.0 ("y") -> [w567]
            n125 = Unbundle By Name(w579) -> ("id"=w575:u32, "function"=w578:T4, "x"=w574:dbl, "y"=w573:dbl)
            n126 = Equal?(x=w578, y=Functions_Enum."Attacker" ("x")) -> (x = y?=w576:bool)
            n127 = case shown="True" w576 {
              tunnel: w575 -> [_ w583]
              tunnel: w574 -> [_ w585]
              tunnel: w573 -> [_ w584]
              tunnel: [w581 w585] -> w570
              tunnel: [w580 w584] -> w569
              tunnel: [w582 w583] -> w572
              tunnel: w571 -> [w582 _]
              tunnel: w568 -> [w581 _]
              tunnel: w567 -> [w580 _]
              frame False {
              }
              frame True {
              }
            }
          }
          n128 = Build Array(w353, w352) -> (w349:dbl[])
          n129 = Build Array(w341, w340) -> (w338:dbl[])
          n130 = Index Array(array=w338) -> (element #1=w336:dbl, element #2=w334:dbl)  [unwired: 2 in]
          n131 = Subtract(x=w335, y=w334) -> (x-y=w332:dbl)
          n132 = Subtract(x=w337, y=w336) -> (x-y=w333:dbl)
          n133 = Build Array(w333, w332) -> (w331:dbl[])
          n134 = call "Modulo.vi"("2D vector"=w331) -> ("Modulo"=w330:dbl)  [unwired: 10 in]
          n135 = Less?(x=w330, y=w327) -> (x < y?=w325:bool)
          n136 = And(x=w312, y=w325) -> (x .and. y?=w317:bool)
          n137 = And(x=w317, y=w318) -> (x .and. y?=w306:bool)
          n138 = case shown="False" w306 {
            tunnel: [w364 FALSE] -> w305
            tunnel: "Dribble" -> [w364 _]
            frame False {
            }
            frame True {
            }
          }
          n139 = case shown="False" w306 {
            tunnel: w362 -> [w418 w462]
            tunnel: w361 -> [w413 w461]
            tunnel: w360 -> [_ w453]
            tunnel: w358 -> [_ w460]
            tunnel: FALSE -> [_ w459]
            tunnel: w349 -> [_ w454]
            tunnel: w347 -> [_ w458]
            tunnel: w346 -> [_ w457]
            tunnel: w315 -> [w419 w450]
            tunnel: w339 -> [w412 w456]
            tunnel: w329 -> [w399 _]
            tunnel: [w398 w455] -> w328
            tunnel: w326 -> [w396 _]
            tunnel: w305 -> [w379 w451]
            tunnel: w313 -> [_ w449]
            frame True {
              # "target"
              # "posição atual\nrobô"
              # "vetor normalizado"
              # "vetor bola->gol"
              # "posição bola"
              # "posição gol"
              n140 = Unbundle By Name(w419) -> ("geometry.field_length"=w420:u32)
              n141 = Index Array(array=w418) -> (element=w424:T8)  [unwired: 1 in]
              n142 = Unbundle By Name(w424) -> ("x"=w393:dbl, "y"=w392:dbl)
              n143 = Unbundle By Name(w412) -> ("x"=w411:dbl, "y"=w410:dbl, "orientation"=w409:dbl)
              n144 = Divide(x=w420, y=u32 2) -> (x/y=w422:dbl)
              n145 = Build Array(w393, w392) -> (w389:dbl[])
              n146 = Multiply(x=w422, y=-1.0) -> (x*y=w395:dbl)
              n147 = Build Array(w411, w410, w409) -> (w408:dbl[])
              n148 = Build Array(w395, 0.0 ("element")) -> (w391:dbl[])
              n149 = Subtract(x=w391, y=w389) -> (x-y=w390:dbl[])
              n150 = call-poly <vilib>:"Vector Norm.vi"("Input Vector"=w390) -> ("norm"=w417:dbl)  [unwired: 9 in, 1 out]
              n151 = Divide(x=w390, y=w417) -> (x/y=w397:dbl[])
              n152 = Multiply(x=w397, y=w396) -> (x*y=w387:dbl[])
              n153 = Index Array(array=w387) -> (element #1=w416:dbl, element #2=w415:dbl)  [unwired: 2 in]
              n154 = Inverse Tangent (2 Input)(1:w416, 2:w415) -> (0:w407:dbl)
              n155 = Add(x=w407, y=3.141592653589793) -> (x+y=w405:dbl)
              n156 = Add(x=w387, y=w389) -> (x+y=w388:dbl[])
              n157 = Insert Into Array(array=w388, index=2, new element=w405) -> (w400:dbl[])
              n158 = case shown="0, Default" w413 {
                tunnel: w408 -> [w427 w430 w433 w436 w439 w442 w445 w448]
                tunnel: w400 -> [w426 w429 w432 w435 w438 w441 w444 w447]
                tunnel: [w425 w428 w431 w434 w437 w440 w443 w446] -> w404
                frame 0, Default {
                  n159 = call "GoTo.vi"("Target"=w426, "Position"=w427) -> ("Output\nVelocity"=w425:dbl[])  [unwired: 8 in, 1 out]
                }
                frame 1 {
                  n160 = call "GoTo.vi"("Target"=w429, "Position"=w430) -> ("Output\nVelocity"=w428:dbl[])  [unwired: 8 in, 1 out]
                }
                frame 2 {
                  n161 = call "GoTo.vi"("Target"=w432, "Position"=w433) -> ("Output\nVelocity"=w431:dbl[])  [unwired: 8 in, 1 out]
                }
                frame 3 {
                  n162 = call "GoTo.vi"("Target"=w435, "Position"=w436) -> ("Output\nVelocity"=w434:dbl[])  [unwired: 8 in, 1 out]
                }
                frame 4 {
                  n163 = call "GoTo.vi"("Target"=w438, "Position"=w439) -> ("Output\nVelocity"=w437:dbl[])  [unwired: 8 in, 1 out]
                }
                frame 5 {
                  n164 = call "GoTo.vi"("Target"=w441, "Position"=w442) -> ("Output\nVelocity"=w440:dbl[])  [unwired: 8 in, 1 out]
                }
                frame 6 {
                  n165 = call "GoTo.vi"("Target"=w444, "Position"=w445) -> ("Output\nVelocity"=w443:dbl[])  [unwired: 8 in, 1 out]
                }
                frame 7 {
                  n166 = call "GoTo.vi"("Target"=w447, "Position"=w448) -> ("Output\nVelocity"=w446:dbl[])  [unwired: 8 in, 1 out]
                }
              }
              n167 = Index Array(array=w404) -> (element #1=w403:dbl, element #2=w402:dbl, element #3=w401:dbl)  [unwired: 3 in]
              n168 = Index Array(array=w400) -> (element #1=w382:dbl, element #2=w381:dbl, element #3=w380:dbl)  [unwired: 3 in]
              n169 = Bundle By Name(cluster=T7 {"dest_x"=0.0, "dest_y"=0.0, "dest_orientation"=0.0, "dest_vel"=0.0} ("Dest"), "dest_x"=w382, "dest_y"=w381, "dest_orientation"=w380, "dest_vel"=0.0) -> (w385:T7)
              n170 = Build Array(w385) -> (w383:T7[])
              n171 = Bundle By Name(cluster=w399, "v_tangent"=w403, "v_normal"=w402, "v_ang"=w401, "Dest"=w383, "dribble"=w379) -> (w398:T3)
            }
            frame False {
              n172 = Select(t=w454, s=w449, f=w453) -> (s? t:f=w452:dbl[])
              n173 = case shown="1" w461 {
                tunnel: w456 -> [w474 w487 w500 w513 w526 w539 w552 w564]
                tunnel: w460 -> [w475 w488 w501 w514 w527 w540 w553 w562]
                tunnel: w462 -> [w473 w486 w499 w512 w525 w538 w551 w566]
                tunnel: w450 -> [w472 w485 w498 w511 w524 w537 w550 w565]
                tunnel: [w471 w484 w497 w510 w523 w536 w549 w563] -> w455
                tunnel: w459 -> [w470 w483 w496 w509 w522 w535 w548 w561]
                tunnel: w458 -> [w469 w482 w495 w508 w521 w534 w547 w560]
                tunnel: w457 -> [w468 w481 w494 w507 w520 w533 w546 w559]
                tunnel: w452 -> [w465 w478 w491 w504 w517 w530 w543 w556]
                tunnel: w451 -> [_ _ _ _ _ _ _ _]
                frame 0, Default {
                  n174 = Unbundle By Name(w468) -> ("Attacker.ball-robot Kick"=w467:dbl, "Attacker.CC chute"=w466:dbl)
                  n175 = call "GoToKick.vi"("goleiro?"=w470, "balls"=w473, "Robot in in"=w474, "Target"=w465, "Field Size in"=w475, "Defender"=TRUE, "D ball - robot"=w467, "AI Parameters"=w468, "Cone de chute"=w466, "Personalidade"=PersonalityEnum."Defender", "Kick Force"=w469, "IA State Input in"=w472) -> ("Robot out"=w471:T3)  [unwired: 12 in, 3 out]
                }
                frame 2 {
                  n176 = Unbundle By Name(w481) -> ("Attacker.ball-robot Kick"=w480:dbl, "Attacker.CC chute"=w479:dbl)
                  n177 = call "GoToKick.vi"("goleiro?"=w483, "balls"=w486, "Robot in in"=w487, "Target"=w478, "Field Size in"=w488, "Defender"=TRUE, "D ball - robot"=w480, "AI Parameters"=w481, "Cone de chute"=w479, "Personalidade"=PersonalityEnum."Defender", "Kick Force"=w482, "IA State Input in"=w485) -> ("Robot out"=w484:T3)  [unwired: 12 in, 3 out]
                }
                frame 3 {
                  n178 = Unbundle By Name(w494) -> ("Attacker.ball-robot Kick"=w493:dbl, "Attacker.CC chute"=w492:dbl)
                  n179 = call "GoToKick.vi"("goleiro?"=w496, "balls"=w499, "Robot in in"=w500, "Target"=w491, "Field Size in"=w501, "Defender"=TRUE, "D ball - robot"=w493, "AI Parameters"=w494, "Cone de chute"=w492, "Personalidade"=PersonalityEnum."Defender", "Kick Force"=w495, "IA State Input in"=w498) -> ("Robot out"=w497:T3)  [unwired: 12 in, 3 out]
                }
                frame 4 {
                  n180 = Unbundle By Name(w507) -> ("Attacker.ball-robot Kick"=w506:dbl, "Attacker.CC chute"=w505:dbl)
                  n181 = call "GoToKick.vi"("goleiro?"=w509, "balls"=w512, "Robot in in"=w513, "Target"=w504, "Field Size in"=w514, "Defender"=TRUE, "D ball - robot"=w506, "AI Parameters"=w507, "Cone de chute"=w505, "Personalidade"=PersonalityEnum."Defender", "Kick Force"=w508, "IA State Input in"=w511) -> ("Robot out"=w510:T3)  [unwired: 12 in, 3 out]
                }
                frame 5 {
                  n182 = Unbundle By Name(w520) -> ("Attacker.ball-robot Kick"=w519:dbl, "Attacker.CC chute"=w518:dbl)
                  n183 = call "GoToKick.vi"("goleiro?"=w522, "balls"=w525, "Robot in in"=w526, "Target"=w517, "Field Size in"=w527, "Defender"=TRUE, "D ball - robot"=w519, "AI Parameters"=w520, "Cone de chute"=w518, "Personalidade"=PersonalityEnum."Defender", "Kick Force"=w521, "IA State Input in"=w524) -> ("Robot out"=w523:T3)  [unwired: 12 in, 3 out]
                }
                frame 6 {
                  n184 = Unbundle By Name(w533) -> ("Attacker.ball-robot Kick"=w532:dbl, "Attacker.CC chute"=w531:dbl)
                  n185 = call "GoToKick.vi"("goleiro?"=w535, "balls"=w538, "Robot in in"=w539, "Target"=w530, "Field Size in"=w540, "Defender"=TRUE, "D ball - robot"=w532, "AI Parameters"=w533, "Cone de chute"=w531, "Personalidade"=PersonalityEnum."Defender", "Kick Force"=w534, "IA State Input in"=w537) -> ("Robot out"=w536:T3)  [unwired: 12 in, 3 out]
                }
                frame 7 {
                  n186 = Unbundle By Name(w546) -> ("Attacker.ball-robot Kick"=w545:dbl, "Attacker.CC chute"=w544:dbl)
                  n187 = call "GoToKick.vi"("goleiro?"=w548, "balls"=w551, "Robot in in"=w552, "Target"=w543, "Field Size in"=w553, "Defender"=TRUE, "D ball - robot"=w545, "AI Parameters"=w546, "Cone de chute"=w544, "Personalidade"=PersonalityEnum."Defender", "Kick Force"=w547, "IA State Input in"=w550) -> ("Robot out"=w549:T3)  [unwired: 12 in, 3 out]
                }
                frame 1 {
                  n188 = Unbundle By Name(w559) -> ("Attacker.ball-robot Kick"=w558:dbl, "Attacker.CC chute"=w557:dbl)
                  n189 = call "GoToKick.vi"("goleiro?"=w561, "balls"=w566, "Robot in in"=w564, "Target"=w556, "Field Size in"=w562, "Defender"=TRUE, "D ball - robot"=w558, "AI Parameters"=w559, "Cone de chute"=w557, "Personalidade"=PersonalityEnum."Defender", "Kick Force"=w560, "IA State Input in"=w565) -> ("Robot out"=w563:T3)  [unwired: 12 in, 3 out]
                }
              }
            }
          }
        }
      }
      n190 = feedback-in #1(w96) -> ()
    }
  }
  "Robot out" <- w8
  "Pos Centers Back" <- w7
